vi "myRIO__TCP_constants_byteRange_numbers__checkRange.vi"(11 "input_byte":u8) -> (0 "output_numbers_negSign":bool, 1 "output_numbers_num":bool, 3 "output_numbers":bool)   [LabVIEW 2014]
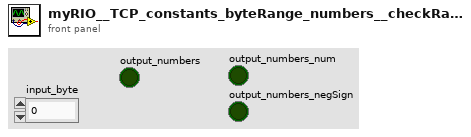
[diagram p1: front panel]
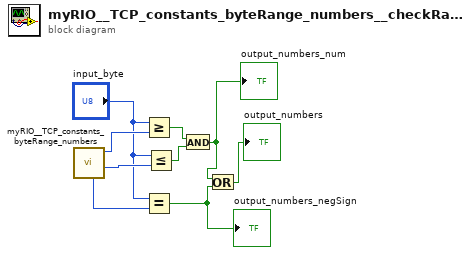
[diagram p0: block diagram]
diagram:
  n1 = call "myRIO__TCP_constants_byteRange_numbers.vi"() -> ("output_byte_end"=w8:u8, "output_byte_start"=w9:u8, "output_byte_negativeSign"=w4:u8)  [unwired: 9 in]
  n2 = Greater Or Equal?(x="input_byte", y=w9) -> (x >= y?=w7:bool)
  n3 = Equal?(x="input_byte", y=w4) -> (x = y?=w3:bool)
  "output_numbers_negSign" <- w3
  n4 = Less Or Equal?(x="input_byte", y=w8) -> (x <= y?=w6:bool)
  n5 = And(x=w7, y=w6) -> (x .and. y?=w2:bool)
  "output_numbers_num" <- w2
  n6 = Or(x=w2, y=w3) -> (x .or. y?=→"output_numbers":bool)
